vi "7-3-1-subvi.vi"(0 "Display Style":u32, 1 "Disabled":T1(ring), 2 "Str Refnum":refnum<vi>, 3 "Bool Refnum":refnum<vi>) -> ()   [LabVIEW 2019]
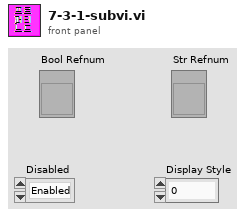
[diagram p1: front panel]
types:
  T1 = enum8{"Enabled", "Disabled", "Disabled and Grayed Out"}
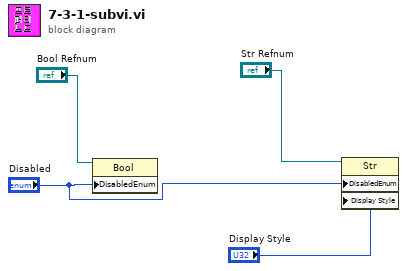
[diagram p0: block diagram]
diagram:
  n1 = property class="Bool"(reference="Bool Refnum", "DisabledEnum"="Disabled") -> ()  [unwired: 1 in, 2 out]
  n2 = property class="Str"(reference="Str Refnum", "DisabledEnum"="Disabled", "Display Style"="Display Style") -> ()  [unwired: 1 in, 2 out]
